vi "Configure External Trigger.vi"(8 "error in (no error)":errorcluster, 9 "Trigger Level (0.0 Volts)":dbl, 10 "Input Impedance (50.0 Ohms)":dbl(ring) items=["50.0", "10000.0"], 11 "VISA resource name":refnum<visa-resource-name>) -> (0 "error out":errorcluster, 3 "VISA resource name out":refnum<visa-resource-name>)   [LabVIEW 2009, in "Agilent 81150.lvlib"]
doc: "Configures the internal trigger source.\n\n<B>Note(s):</B>\n(1) This is applicable when the <B>Trigger Source</B> is set to external."
uses:
  Agilent 81150.lvlib
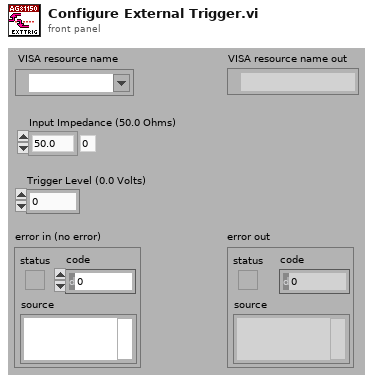
[diagram p1: front panel]
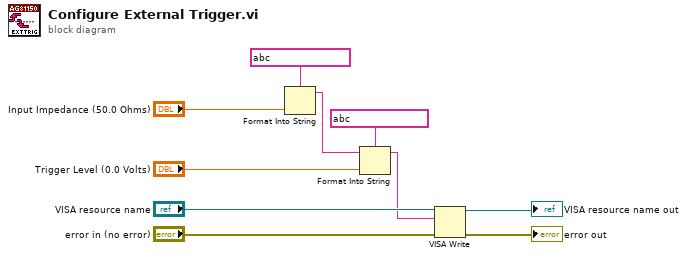
[diagram p0: block diagram]
diagram:
  n1 = Format Into String(format string=string ?, "Input Impedance (50.0 Ohms)") -> (resulting string=w8:string)  [unwired: 2 in, 1 out]
  n2 = Format Into String(format string=string ?, initial string=w8, "Trigger Level (0.0 Volts)") -> (resulting string=w1:string)  [unwired: 1 in, 1 out]
  n3 = VISA Write(VISA resource name="VISA resource name", write buffer=w1, error in (no error)="error in (no error)") -> (VISA resource name out=→"VISA resource name out":refnum<visa-resource-name>, error out=→"error out":errorcluster)  [unwired: 1 out]
